vi "Triax320 GetStepPos.vi"(8 "error in (no error)":errorcluster, 11 "Triax VISA Rsrc":refnum<visa-resource-name>="SR530") -> (0 "error out":errorcluster, 2 "Step Out":u32=100 caption="Longueur d'ondes(nm)", 3 "Triax VISA Rsrc Out":refnum<visa-resource-name>="SR530")   [LabVIEW 2019]
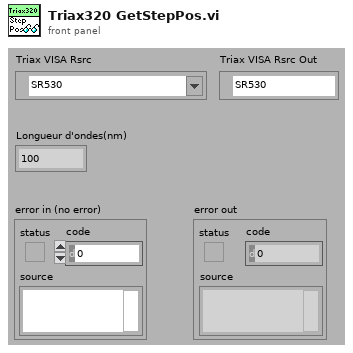
[diagram p1: front panel]
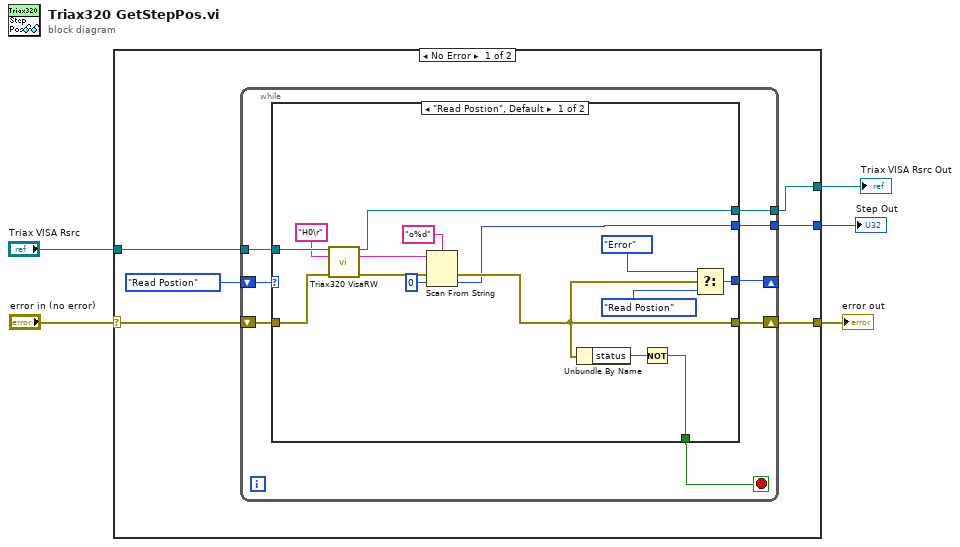
[diagram p0: block diagram]
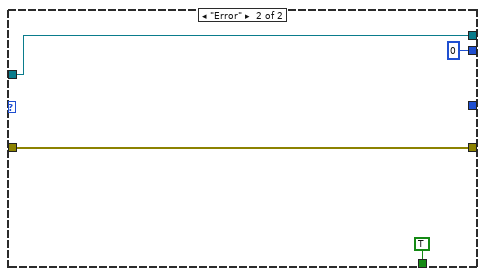
[diagram p2: hidden frame]
diagram:
  n1 = case shown="No Error" "error in (no error)" {
    selector: "error in (no error)" -> [w10 w40]
    tunnel: "Triax VISA Rsrc" -> [w11 w39]
    tunnel: [w8 w40] -> w3
    tunnel: [w7 _] -> w2
    tunnel: [w6 w39] -> w1
    frame No Error {
      n2 = while {
        shift-right: [w17] -> _
        shift-left: enum16{"Error", "Read Postion"}."Read Postion" -> [w19]
        tunnel: w11 -> [w16]
        shift-right: [w14] -> w8
        shift-left: w10 -> [w15]
        tunnel: [w13] -> w6
        tunnel: [w12] -> w7
        stop <- w18 stop-if-true
        n3 = case shown="\"Read Postion\", Default" w19 {
          tunnel: [w23 TRUE] -> w18
          tunnel: [w30 _] -> w17
          tunnel: w16 -> [w34 w38]
          tunnel: w15 -> [w33 w36]
          tunnel: [w22 w36] -> w14
          tunnel: [w32 w38] -> w13
          tunnel: [w21 u32 0] -> w12
          frame "Read Postion", Default {
            n4 = call <userlib>:"Triax320 VisaRW.vi"("VISA Rsrc"=w34, "ChaineCom"="H0\r" ("chaîne"), "error in (no error)"=w33) -> ("VISA Rsrc Out"=w32:refnum<visa-resource-name>, "ChaineRep"=w29:string, "error out"=w27:errorcluster)  [unwired: 7 in, 3 out]
            n5 = Scan From String(format string="o%d" ("chaîne de format"), input string=w29, error in=w27, default 1=u32 0 ("valeur par défaut 1")) -> (error out=w22:errorcluster, output 1=w21:u32)  [unwired: 1 in, 2 out]
            n6 = Unbundle By Name(w22) -> ("status"=w24:bool)
            n7 = Not(x=w24) -> (.not. x?=w23:bool)
            n8 = Select(t=enum16{"Error", "Read Postion"}."Error", s=w22, f=enum16{"Error", "Read Postion"}."Read Postion") -> (s? t:f=w30:enum16{"Error", "Read Postion"})
          }
          frame "Error" {
          }
        }
      }
    }
    frame Error {
    }
  }
  "error out" <- w3
  "Step Out" <- w2
  "Triax VISA Rsrc Out" <- w1
